vi "Destroy.vi"(0 "reference in":refnum<class "Object.lvclass">, 5 "error in (no error)":errorcluster) -> (14 "reference out":refnum<class "Object.lvclass">, 19 "error out":errorcluster)   [LabVIEW 2020, in "Object.lvclass"]
doc: "Destroys the object and stops the walkabout process"
uses:
  Object.lvclass
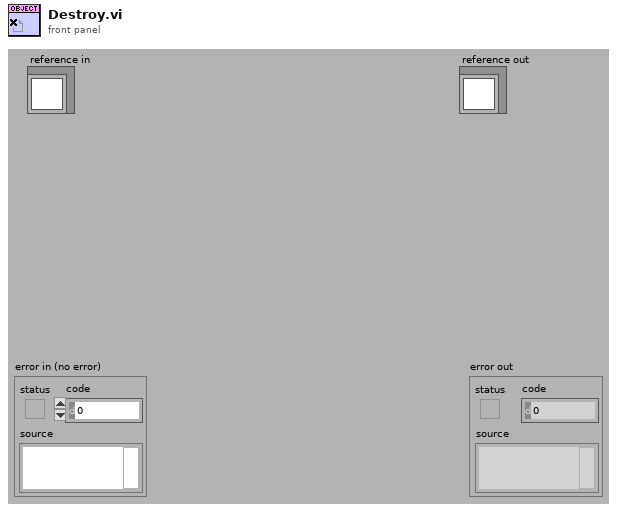
[diagram p1: front panel]
types:
  T1 = typedef "Object.lvclass/ClassAttributes.ctl" = cluster{"Objects":i32}
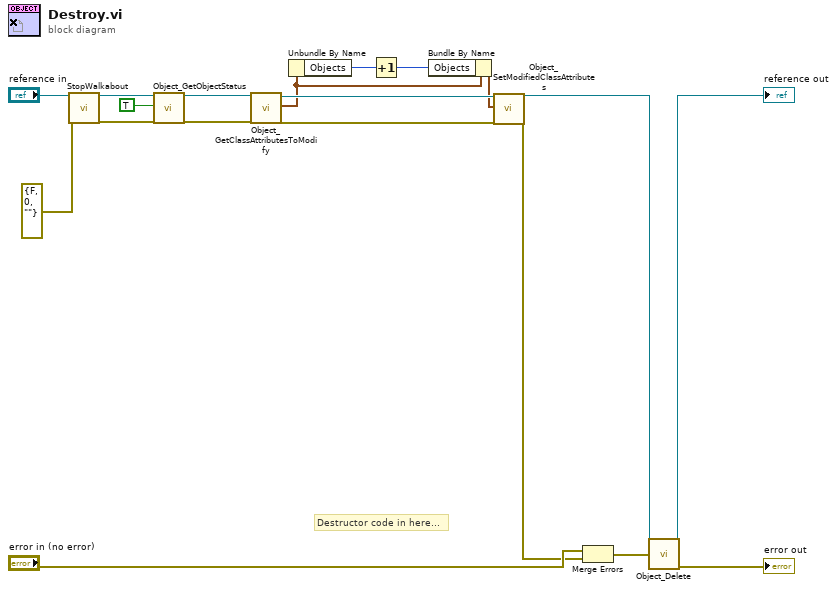
[diagram p0: block diagram]
diagram:
  # "Destructor code in here..."
  n1 = call "StopWalkabout.vi"("reference in"="reference in", "error in (no error)"=errorcluster {"status"=FALSE, "code"=0, "source"=""}) -> ("reference out"=w12:refnum<class "Object.lvclass">, "error out"=w2:errorcluster)  [unwired: 1 in, 15 out]
  n2 = call "Object_GetObjectStatus.vi"("reference in"=w12, "Simple Info"=TRUE, "error in (no error)"=w2) -> ("reference out"=w4:refnum<class "Object.lvclass">, "error out"=w5:errorcluster)  [unwired: 15 out]
  n3 = call "Object_GetClassAttributesToModify.vi"("reference in"=w4, "error in (no error)"=w5) -> ("reference out"=w11:refnum<class "Object.lvclass">, "Class attributes"=w8:T1, "error out"=w10:errorcluster)  [unwired: 1 in, 14 out]
  n4 = Unbundle By Name(w8) -> ("Objects"=w9:i32)
  n5 = Increment(x=w9) -> (x+1=w6:i32)
  n6 = Bundle By Name(cluster=w8, "Objects"=w6) -> (w7:T1)
  n7 = call "Object_SetModifiedClassAttributes.vi"("reference in"=w11, "Class attributes"=w7, "error in (no error)"=w10) -> ("error out"=w1:errorcluster)  [unwired: 2 in, 14 out]
  n8 = Merge Errors("error in (no error)", w1) -> (w16:errorcluster)
  n9 = call "Object_Delete.vi"("reference in"=w4, "error in (no error)"=w16) -> ("reference out"=→"reference out":refnum<class "Object.lvclass">, "error out"=→"error out":errorcluster)  [unwired: 1 in, 15 out]
